vi "RTD Temp.vi"(0 "error in (no error)":errorcluster) -> (1 "RTD Temp":dbl(slide) scale=0.0..100.0, 2 "error out":errorcluster)   [LabVIEW 2024]
uses:
  <vilib>/Utility/error.llb/DialogType.ctl
  <vilib>/DAQmx/read.llb/DAQmx Read (Analog 1D DBL 1Chan NSamp).vi
  <vilib>/Analysis/baseanly.llb/Mean (DBL).vi
  <vilib>/DAQmx/create/channels.llb/DAQmx Create Channel (AI-Voltage-Basic).vi
  <vilib>/DAQmx/configure/timing.llb/DAQmx Timing (Sample Clock).vi
  <vilib>/DAQmx/miscellaneous.llb/DAQmx Fill In Error Info.vi
  <vilib>/Analysis/NI_AALBase.lvlib
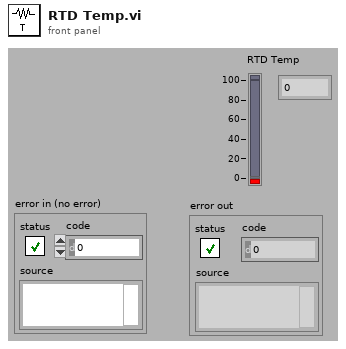
[diagram p1: front panel]
types:
  T1 = typedef "DialogType.ctl" = u16
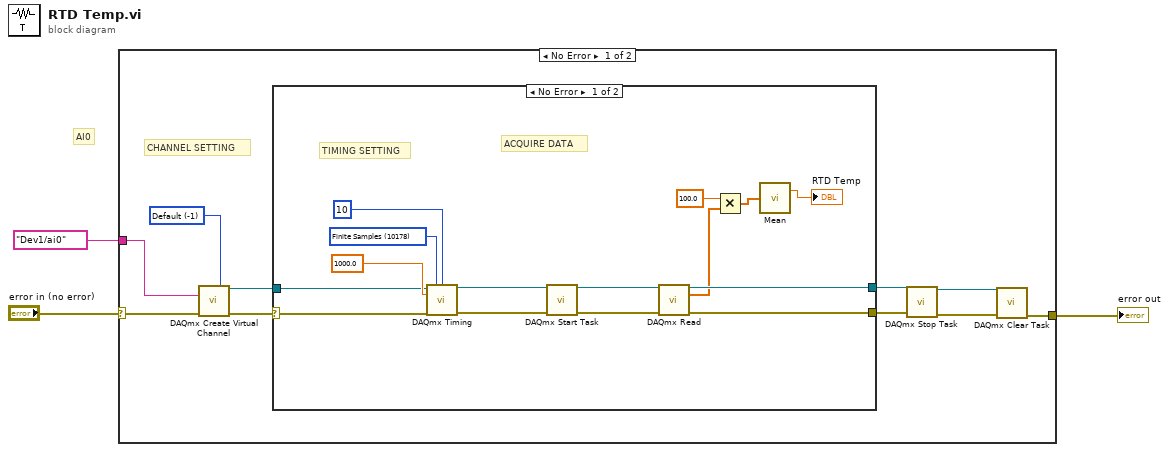
[diagram p0: block diagram]
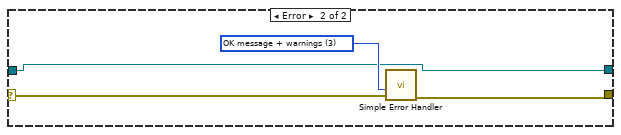
[diagram p2: hidden frame]
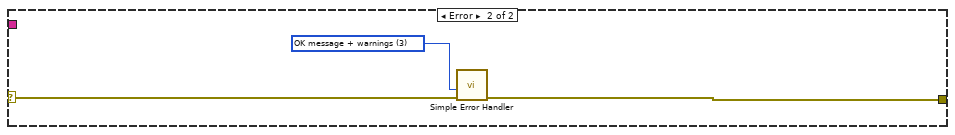
[diagram p3: hidden frame]
diagram:
  # "AI0"
  n1 = case shown="No Error" "error in (no error)" {
    selector: "error in (no error)" -> [w13 w34]
    tunnel: tag "Dev1/ai0" ("physical channels") -> [w11 _]
    tunnel: [w6 w33] -> w2
    frame No Error {
      w10 = -1 items=["Default"=-1, "RSE"=10083, "NRSE"=10078, "Differential"=10106, "Pseudodifferential"=12529] ("input terminal configuration")
      # "CHANNEL SETTING"
      n2 = call-poly <vilib>:"DAQmx Create Virtual Channel.vi"("input terminal configuration"=w10, "physical channels"=w11, "error in"=w13) -> ("task out"=w9:refnum<k21>, "error out"=w12:errorcluster)  [unwired: 11 in]
      n3 = case shown="No Error" w12 {
        selector: w12 -> [w21 w31]
        tunnel: w9 -> [w20 w29]
        tunnel: [w19 w30] -> w5
        tunnel: [w18 w29] -> w4
        frame No Error {
          w28 = 10178 items=["Finite Samples"=10178, "Continuous Samples"=10123, "Hardware Timed Single Point"=12522] ("sample mode")
          # "ACQUIRE DATA"
          # "TIMING SETTING"
          n4 = call-poly <vilib>:"DAQmx Timing.vi"("task/channels in"=w20, "sample mode"=w28, "samples per channel"=10, "rate"=1000.0, "error in"=w21) -> ("task out"=w25:refnum<k21>, "error out"=w24:errorcluster)  [unwired: 9 in]
          n5 = call <vilib>:"DAQmx Start Task.vi"("task/channels in"=w25, "error in"=w24) -> ("task out"=w23:refnum<k21>, "error out"=w22:errorcluster)  [unwired: 12 in]
          n6 = call-poly <vilib>:"DAQmx Read.vi"("task/channels in"=w23, "error in"=w22) -> ("task out"=w18:refnum<k21>, "data"=w16:dbl[], "error out"=w19:errorcluster)  [unwired: 11 in]
          n7 = Multiply(x=100.0, y=w16) -> (x*y=w15:dbl[])
          n8 = call-poly <vilib>:"Mean.vi"("X"=w15) -> ("mean"=→"RTD Temp":dbl)  [unwired: 1 out]
        }
        frame Error {
          w32 = T1 3 items=["no dialog", "OK message", "continue or stop message", "OK message + warnings", "continue/stop + warnings"] ("type of dialog (OK msg:1)")
          n9 = call <vilib>:"Simple Error Handler.vi"("type of dialog (OK msg:1)"=w32, "error in (no error)"=w31) -> ("error out"=w30:errorcluster)  [unwired: 3 in, 4 out]
        }
      }
      n10 = call <vilib>:"DAQmx Stop Task.vi"("task/channels in"=w4, "error in"=w5) -> ("task out"=w7:refnum<k21>, "error out"=w8:errorcluster)  [unwired: 12 in]
      n11 = call <vilib>:"DAQmx Clear Task.vi"("task in"=w7, "error in"=w8) -> ("error out"=w6:errorcluster)  [unwired: 13 in]
    }
    frame Error {
      w35 = T1 3 items=["no dialog", "OK message", "continue or stop message", "OK message + warnings", "continue/stop + warnings"] ("type of dialog (OK msg:1)")
      n12 = call <vilib>:"Simple Error Handler.vi"("type of dialog (OK msg:1)"=w35, "error in (no error)"=w34) -> ("error out"=w33:errorcluster)  [unwired: 3 in, 4 out]
    }
  }
  "error out" <- w2
